vi "VG_OCV30max_P.vi"() -> ()   [LabVIEW 2020]
panel:
  out "OCV30max":dbl
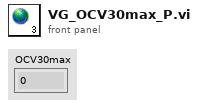
[diagram p1: front panel]
diagram:
